vi "ReadCluster.vi"(1 "reference":refnum<vi>) -> (0 "Cluster":T6)   [LabVIEW 2013]
uses:
  <vilib>/Utility/miscctls.llb/LVBoundsTypeDef.ctl
  <vilib>/Utility/miscctls.llb/LVRectTypeDef.ctl
  <vilib>/Utility/miscctls.llb/LVPositionTypeDef.ctl
  <vilib>/Utility/miscctls.llb/LVDataSocketStatusTypeDef.ctl
  <vilib>/Utility/miscctls.llb/LVKeyNavTypeDef.ctl
panel:
  out "error out":errorcluster
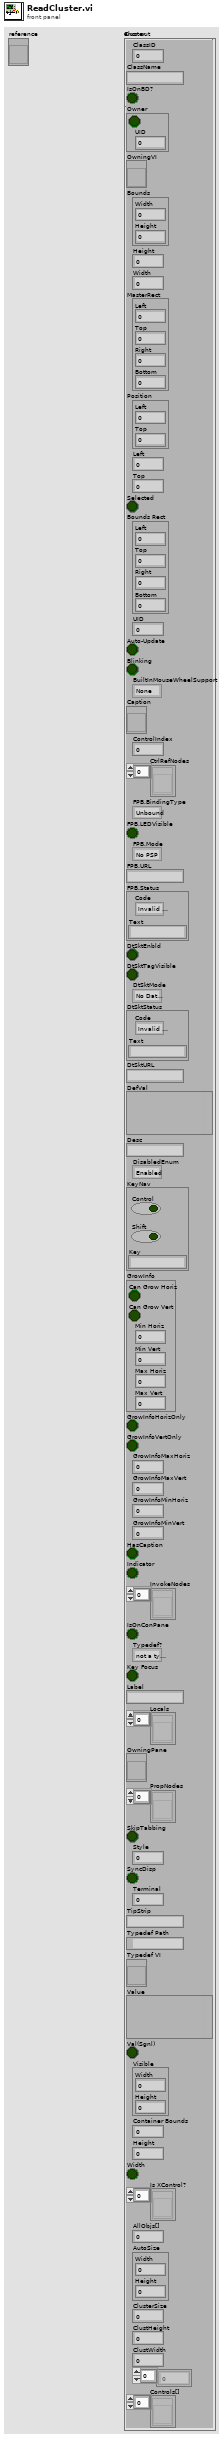
[diagram p1: front panel]
types:
  T1 = typedef "LVBoundsTypeDef.ctl" = cluster{"Width":u32, "Height":u32}
  T2 = typedef "LVRectTypeDef.ctl" = cluster{"Left":i16, "Top":i16, "Right":i16, "Bottom":i16}
  T3 = typedef "LVPositionTypeDef.ctl" = cluster{"Left":i32, "Top":i32}
  T4 = typedef "LVDataSocketStatusTypeDef.ctl" = cluster{"Code":enum32{"Invalid Status", "Unconnected", "Active", "Idle", "Error", "Connecting"}, "Text":string}
  T5 = typedef "LVKeyNavTypeDef.ctl" = cluster{"Control":bool, "Shift":bool, "Key":string}
  T6 = cluster{"ClassID":u32, "ClassName":string, "IsOnBD?":bool, "Owner":cluster{bool, "UID":i32}, "OwningVI":refnum<vi>, "Bounds":T1, "Height":u32, "Width":u32, "MasterRect":T2, "Position":T3, "Left":i32, "Top":i32, "Selected":bool, "Bounds Rect":T2, "UID":i32, "Auto-Update":bool, "Blinking":bool, "BuiltInMouseWheelSupport":enum16{"None", "On Hover", "On Key Focus", "On Hover or Key Focus"}, "Caption":refnum<vi>, "ControlIndex":i32, "CtrlRefNodes":refnum<vi>[], "FPB.BindingType":enum32{"Unbound", "Bound To PSP URL", "Bound To Variable Shortcut"}, "FPB.LEDVisible":bool, "FPB.Mode":enum32{"No PSP", "Read", "Write", "Write & Read"}, "FPB.URL":string, "FPB.Status":T4, "DtSktEnbld":bool, "DtSktTagVisible":bool, "DtSktMode":enum32{"No DataSocket", "Publish", "Subscribe", "Publish & Subscribe"}, "DtSktStatus":T4, "DtSktURL":string, "DefVal":variant, "Desc":string, "DisabledEnum":enum8{"Enabled", "Disabled", "Disabled and Grayed Out"}, "KeyNav":T5, "GrowInfo":cluster{"Can Grow Horiz":bool, "Can Grow Vert":bool, "Min Horiz":i16, "Min Vert":i16, "Max Horiz":i16, "Max Vert":i16}, "GrowInfoHorizOnly":bool, "GrowInfoVertOnly":bool, "GrowInfoMaxHoriz":i16, "GrowInfoMaxVert":i16, "GrowInfoMinHoriz":i16, "GrowInfoMinVert":i16, "HasCaption":bool, "Indicator":bool, "InvokeNodes":refnum<vi>[], "IsOnConPane":bool, "Typedef?":enum32{"not a typedef", "typedef", "strict typedef", "class private data"}, "Key Focus":bool, "Label":string, "Locals":refnum<vi>[], "OwningPane":refnum<vi>, "PropNodes":refnum<vi>[], "SkipTabbing":bool, "Style":u32, "SyncDisp":bool, "Terminal":i32, "TipStrip":string, "Typedef Path":path, "Typedef VI":refnum<vi>, "Value":variant, "Val(Sgnl)":bool, "Visible":T1, "Container Bounds":u32, "Height":u32, "Width":bool, "Is XControl?":refnum<vi>[], "AllObjs[]":u32, "AutoSize":T1, "ClusterSize":u32, "ClustHeight":u32, "ClustWidth":u32, "Color":i32[], "Controls[]":refnum<vi>[]}
  T7 = enum16{"None", "On Hover", "On Key Focus", "On Hover or Key Focus"}
  T8 = enum32{"Unbound", "Bound To PSP URL", "Bound To Variable Shortcut"}
  T9 = enum32{"No PSP", "Read", "Write", "Write & Read"}
  T10 = enum32{"No DataSocket", "Publish", "Subscribe", "Publish & Subscribe"}
  T11 = enum8{"Enabled", "Disabled", "Disabled and Grayed Out"}
  T12 = cluster{"Can Grow Horiz":bool, "Can Grow Vert":bool, "Min Horiz":i16, "Min Vert":i16, "Max Horiz":i16, "Max Vert":i16}
  T13 = enum32{"not a typedef", "typedef", "strict typedef", "class private data"}
  T14 = cluster{"ClassID":u32, "ClassName":string, "IsOnBD?":bool, "Cluster":cluster{bool, "UID":i32}, "OwningVI":refnum<vi>, "Bounds":T1, "Height":u32, "Width":u32, "MasterRect":T2, "Position":T3, "Left":i32, "Top":i32, "Selected":bool, "Bounds Rect":T2, "UID":i32, "Auto-Update":bool, "Blinking":bool, "BuiltInMouseWheelSupport":enum16{"None", "On Hover", "On Key Focus", "On Hover or Key Focus"}, "Caption":refnum<vi>, "ControlIndex":i32, "CtrlRefNodes":refnum<vi>[], "FPB.BindingType":enum32{"Unbound", "Bound To PSP URL", "Bound To Variable Shortcut"}, "FPB.LEDVisible":bool, "FPB.Mode":enum32{"No PSP", "Read", "Write", "Write & Read"}, "FPB.URL":string, "FPB.Status":T4, "DtSktEnbld":bool, "DtSktTagVisible":bool, "DtSktMode":enum32{"No DataSocket", "Publish", "Subscribe", "Publish & Subscribe"}, "DtSktStatus":T4, "DtSktURL":string, "DefVal":variant, "Desc":string, "DisabledEnum":enum8{"Enabled", "Disabled", "Disabled and Grayed Out"}, "KeyNav":T5, "GrowInfo":cluster{"Can Grow Horiz":bool, "Can Grow Vert":bool, "Min Horiz":i16, "Min Vert":i16, "Max Horiz":i16, "Max Vert":i16}, "GrowInfoHorizOnly":bool, "GrowInfoVertOnly":bool, "GrowInfoMaxHoriz":i16, "GrowInfoMaxVert":i16, "GrowInfoMinHoriz":i16, "GrowInfoMinVert":i16, "HasCaption":bool, "Indicator":bool, "InvokeNodes":refnum<vi>[], "IsOnConPane":bool, "Typedef?":enum32{"not a typedef", "typedef", "strict typedef", "class private data"}, "Key Focus":bool, "Text":string, "Locals":refnum<vi>[], "OwningPane":refnum<vi>, "PropNodes":refnum<vi>[], "SkipTabbing":bool, "Style":u32, "SyncDisp":bool, "UID":i32, "TipStrip":string, "Typedef Path":path, "Typedef VI":refnum<vi>, "Value":variant, "Visible":bool, "Container Bounds":T1, "Height":u32, "Width":u32, "Is XControl?":bool, "AllObjs[]":refnum<vi>[], "AutoSize":u32, "ClusterSize":T1, "ClustHeight":u32, "ClustWidth":u32, "Color":u32, i32[], "Decos[]":refnum<vi>[]}
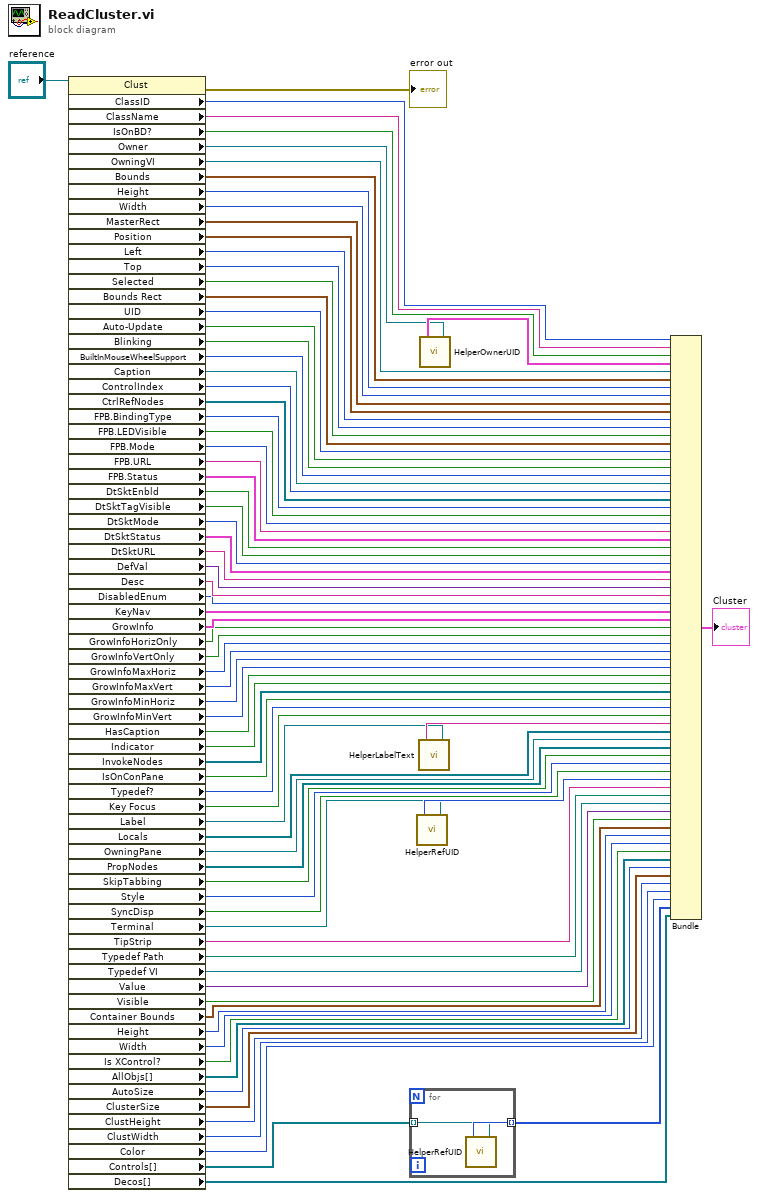
[diagram p0: block diagram]
diagram:
  n1 = property class="Clust"(reference="reference") -> (error out=→"error out":errorcluster, "ClassID"=w78:u32, "ClassName"=w77:string, "IsOnBD?"=w76:bool, "Owner"=w74:refnum<vi>, "OwningVI"=w73:refnum<vi>, "Bounds"=w72:T1, "Height"=w71:u32, "Width"=w70:u32, "MasterRect"=w69:T2, "Position"=w68:T3, "Left"=w67:i32, "Top"=w66:i32, "Selected"=w65:bool, "Bounds Rect"=w64:T2, "UID"=w63:i32, "Auto-Update"=w62:bool, "Blinking"=w61:bool, "BuiltInMouseWheelSupport"=w60:T7, "Caption"=w59:refnum<vi>, "ControlIndex"=w58:i32, "CtrlRefNodes"=w57:refnum<vi>[], "FPB.BindingType"=w56:T8, "FPB.LEDVisible"=w55:bool, "FPB.Mode"=w54:T9, "FPB.URL"=w53:string, "FPB.Status"=w52:T4, "DtSktEnbld"=w51:bool, "DtSktTagVisible"=w50:bool, "DtSktMode"=w49:T10, "DtSktStatus"=w48:T4, "DtSktURL"=w47:string, "DefVal"=w46:variant, "Desc"=w45:string, "DisabledEnum"=w44:T11, "KeyNav"=w43:T5, "GrowInfo"=w42:T12, "GrowInfoHorizOnly"=w41:bool, "GrowInfoVertOnly"=w40:bool, "GrowInfoMaxHoriz"=w39:i16, "GrowInfoMaxVert"=w38:i16, "GrowInfoMinHoriz"=w37:i16, "GrowInfoMinVert"=w36:i16, "HasCaption"=w35:bool, "Indicator"=w34:bool, "InvokeNodes"=w33:refnum<vi>[], "IsOnConPane"=w32:bool, "Typedef?"=w31:T13, "Key Focus"=w30:bool, "Label"=w28:refnum<vi>, "Locals"=w27:refnum<vi>[], "OwningPane"=w26:refnum<vi>, "PropNodes"=w25:refnum<vi>[], "SkipTabbing"=w24:bool, "Style"=w23:u32, "SyncDisp"=w22:bool, "Terminal"=w20:refnum<vi>, "TipStrip"=w19:string, "Typedef Path"=w18:path, "Typedef VI"=w17:refnum<vi>, "Value"=w16:variant, "Visible"=w15:bool, "Container Bounds"=w14:T1, "Height"=w13:u32, "Width"=w12:u32, "Is XControl?"=w11:bool, "AllObjs[]"=w10:refnum<vi>[], "AutoSize"=w9:u32, "ClusterSize"=w8:T1, "ClustHeight"=w7:u32, "ClustWidth"=w6:u32, "Color"=w5:u32, "Controls[]"=w3:refnum<vi>[], "Decos[]"=w2:refnum<vi>[])  [unwired: 1 in, 1 out]
  n2 = for {
    tunnel: [w82] -> w4 mode=indexing
    tunnel: w3 -> [w81] mode=indexing
    n3 = call "HelperRefUID.vi"("Text in"=w81) -> ("UID"=w82:i32)
  }
  n4 = call "HelperRefUID.vi"("Text in"=w20) -> ("UID"=w21:i32)
  n5 = call "HelperLabelText.vi"("Text in"=w28) -> ("Text"=w29:string)
  n6 = call "HelperOwnerUID.vi"("Generic in"=w74) -> ("Cluster"=w75:cluster{bool, "UID":i32})
  n7 = Bundle("ClassID"=w78, "ClassName"=w77, "IsOnBD?"=w76, "Cluster"=w75, "OwningVI"=w73, "Bounds"=w72, "Height"=w71, "Width"=w70, "MasterRect"=w69, "Position"=w68, "Left"=w67, "Top"=w66, "Selected"=w65, "Bounds Rect"=w64, "UID"=w63, "Auto-Update"=w62, "Blinking"=w61, "BuiltInMouseWheelSupport"=w60, "Caption"=w59, "ControlIndex"=w58, "CtrlRefNodes"=w57, "FPB.BindingType"=w56, "FPB.LEDVisible"=w55, "FPB.Mode"=w54, "FPB.URL"=w53, "FPB.Status"=w52, "DtSktEnbld"=w51, "DtSktTagVisible"=w50, "DtSktMode"=w49, "DtSktStatus"=w48, "DtSktURL"=w47, "DefVal"=w46, "Desc"=w45, "DisabledEnum"=w44, "KeyNav"=w43, "GrowInfo"=w42, "GrowInfoHorizOnly"=w41, "GrowInfoVertOnly"=w40, "GrowInfoMaxHoriz"=w39, "GrowInfoMaxVert"=w38, "GrowInfoMinHoriz"=w37, "GrowInfoMinVert"=w36, "HasCaption"=w35, "Indicator"=w34, "InvokeNodes"=w33, "IsOnConPane"=w32, "Typedef?"=w31, "Key Focus"=w30, "Text"=w29, "Locals"=w27, "OwningPane"=w26, "PropNodes"=w25, "SkipTabbing"=w24, "Style"=w23, "SyncDisp"=w22, "UID"=w21, "TipStrip"=w19, "Typedef Path"=w18, "Typedef VI"=w17, "Value"=w16, "Visible"=w15, "Container Bounds"=w14, "Height"=w13, "Width"=w12, "Is XControl?"=w11, "AllObjs[]"=w10, "AutoSize"=w9, "ClusterSize"=w8, "ClustHeight"=w7, "ClustWidth"=w6, "Color"=w5, w4, "Decos[]"=w2) -> (→"Cluster":T14)  [unwired: 1 in]
